vi "Global Stop.vi"(7 "Command":T1=enum."Read", 8 "error in (no error)":errorcluster, 9 "Stop on Error?":bool=TRUE, 10 "Stop?":bool) -> (0 "error out":errorcluster, 1 "Skipped?":bool=TRUE, 2 "Latched Stop":bool)   [LabVIEW 2014, in "Waveform-Processing-Custom-Device Engine.lvlib" / "Stop FG.lvlib"]
uses:
  Stop FG.lvlib
  Stop Global Commands.ctl
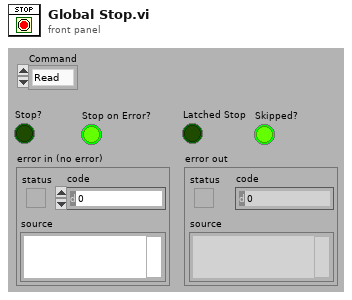
[diagram p1: front panel]
types:
  T1 = typedef "Waveform-Processing-Custom-Device Engine.lvlib/Stop FG.lvlib/Stop Global Commands.ctl" = enum16{"Write", "Read", "Reset"}
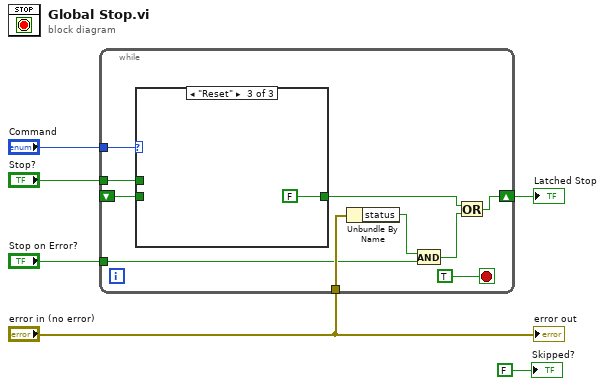
[diagram p0: block diagram]
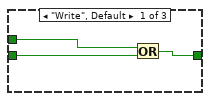
[diagram p2: hidden frame]
diagram:
  n1 = while {
    shift-right: [w12] -> w3
    shift-left: _ -> [w15]
    tunnel: "Stop?" -> [w14]
    tunnel: "Command" -> [w13]
    tunnel: "error in (no error)" -> [w10]
    tunnel: "Stop on Error?" -> [w7]
    stop <- TRUE stop-if-true
    n2 = case shown="\"Reset\"" w13 {
      tunnel: w15 -> [w19 w20 _]
      tunnel: [w17 w20 FALSE ("Stop?")] -> w11
      tunnel: w14 -> [w18 _ _]
      frame "Write", Default {
        n3 = Or(x=w18, y=w19) -> (x .or. y?=w17:bool)
      }
      frame "Read" {
      }
      frame "Reset" {
      }
    }
    n4 = Unbundle By Name(w10) -> ("status"=w9:bool)
    n5 = And(x=w9, y=w7) -> (x .and. y?=w8:bool)
    n6 = Or(x=w11, y=w8) -> (x .or. y?=w12:bool)
  }
  "Latched Stop" <- w3
  "error out" <- "error in (no error)"
  "Skipped?" <- FALSE ("Skipped?")
